vi "RobotLineDest.vi"(10 "Average Distance":dbl, 11 "Angle":dbl) -> ()   [LabVIEW 2013]
uses:
  <vilib>/Rock Robotics/WPI/DriverStation/WPI_DriverStationAllianceInfo.ctl
  <vilib>/Rock Robotics/Network Tables/SD Write Number.vi
  Robot Global Data.vi
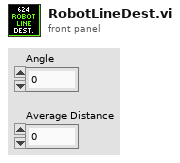
[diagram p1: front panel]
types:
  T1 = typedef "WPI_DriverStationAllianceInfo.ctl" = enum16{"Red", "Blue", "Invalid"}
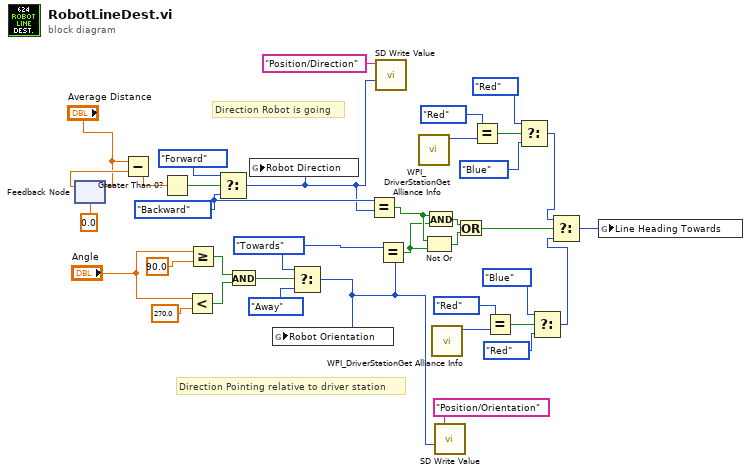
[diagram p0: block diagram]
diagram:
  w31 = enum16{"Forward", "Backward"}."Backward" ("f")
  w32 = enum16{"Away", "Towards"}."Towards" ("y")
  # "Direction Robot is going"
  # "Direction Pointing relative to driver station"
  n1 = feedback-in #1("Average Distance") -> ()
  n2 = feedback #1(0.0 ("Average Distance")) -> (w21:dbl)
  n3 = Subtract(x="Average Distance", y=w21) -> (x-y=w19:dbl)
  n4 = Greater Than 0?(x=w19) -> (x > 0?=w29:bool)
  n5 = Less?(x="Angle", y=270.0) -> (x < y?=w25:bool)
  n6 = Greater Or Equal?(x="Angle", y=90.0) -> (x >= y?=w26:bool)
  n7 = Select(t=enum16{"Forward", "Backward"}."Forward" ("Robot Direction"), s=w29, f=w31) -> (s? t:f=w5:enum16{"Forward", "Backward"})
  n8 = And(x=w26, y=w25) -> (x .and. y?=w27:bool)
  n9 = global write "Robot Global Data.vi" "Robot Direction"(w5) -> ()
  n10 = Select(t=w32, s=w27, f=enum16{"Away", "Towards"}."Away" ("y")) -> (s? t:f=w2:enum16{"Away", "Towards"})
  n11 = global write "Robot Global Data.vi" "Robot Orientation"(w2) -> ()
  n12 = Equal?(x=w5, y=w31) -> (x = y?=w33:bool)
  n13 = call-poly <vilib>:"SD Write Value.vi"("Numeric"=w5, "Name"="Position/Direction") -> ()  [unwired: 8 in, 2 out]
  n14 = Equal?(x=w32, y=w2) -> (x = y?=w1:bool)
  n15 = call <vilib>:"WPI_DriverStationGet Alliance Info.vi"() -> ("Alliance"=w17:T1)  [unwired: 10 in, 1 out]
  n16 = Not Or(1:w1, 2:w33) -> (0:w35:bool)
  n17 = And(x=w33, y=w1) -> (x .and. y?=w34:bool)
  n18 = call <vilib>:"WPI_DriverStationGet Alliance Info.vi"() -> ("Alliance"=w8:T1)  [unwired: 10 in, 1 out]
  n19 = call-poly <vilib>:"SD Write Value.vi"("Numeric"=w2, "Name"="Position/Orientation") -> ()  [unwired: 8 in, 2 out]
  n20 = Or(x=w34, y=w35) -> (x .or. y?=w36:bool)
  n21 = Equal?(x=WPI_DriverStationAllianceInfo."Red", y=w17) -> (x = y?=w15:bool)
  n22 = Equal?(x=WPI_DriverStationAllianceInfo."Red", y=w8) -> (x = y?=w10:bool)
  n23 = Select(t=enum16{"Red", "Blue"}."Red" ("f"), s=w15, f=enum16{"Red", "Blue"}."Blue" ("Line Heading Towards")) -> (s? t:f=w6:enum16{"Red", "Blue"})
  n24 = Select(t=enum16{"Red", "Blue"}."Blue" ("f"), s=w10, f=enum16{"Red", "Blue"}."Red" ("Line Heading Towards")) -> (s? t:f=w7:enum16{"Red", "Blue"})
  n25 = Select(t=w6, s=w36, f=w7) -> (s? t:f=w37:enum16{"Red", "Blue"})
  n26 = global write "Robot Global Data.vi" "Line Heading Towards"(w37) -> ()
